vi "ImageAquisition.vi"() -> ()   [LabVIEW 2021]
uses:
  <vilib>/userdefined/High Color/IMAQdx.ctl
  <vilib>/vision/driver/IMAQdx.llb/IMAQdx Acquisition Mode.ctl
  <vilib>/vision/driver/IMAQdx.llb/IMAQdx Buffer Number Mode.ctl
  <vilib>/vision/driver/IMAQdx.llb/IMAQdx Camera Control Mode.ctl
  <vilib>/vision/driver/NI_Vision_Acquisition_Software.lvlib
panel:
  out "Image":T1(plugin-control)
  in  "Session In":T2="4kCam"
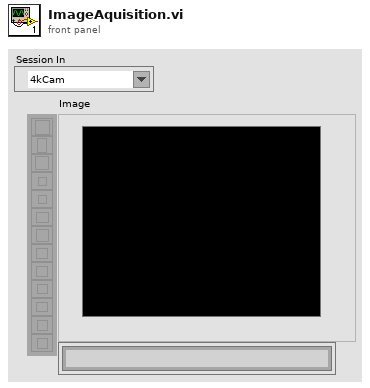
[diagram p1: front panel]
types:
  T1 = typedef "IMAQ Image.ctl" = refnum<image>
  T2 = typedef "IMAQdx.ctl" = refnum<k21>
  T3 = typedef "Image Type" = u32
  T4 = typedef "NI_Vision_Acquisition_Software.lvlib/IMAQdx Camera Control Mode.ctl" = enum32{"Controller", "Listener"}
  T5 = typedef "NI_Vision_Acquisition_Software.lvlib/IMAQdx Buffer Number Mode.ctl" = enum32{"Next", "Last", "Buffer Number", "Every", "Last New"}
  T6 = typedef "NI_Vision_Acquisition_Software.lvlib/IMAQdx Acquisition Mode.ctl" = enum32{"One Shot", "Continuous"}
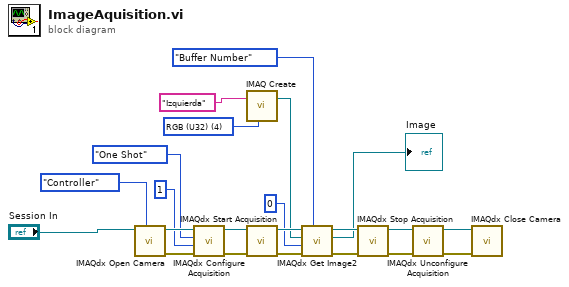
[diagram p0: block diagram]
diagram:
  w3 = T3 4 items=["Grayscale (U8)", "Grayscale (I16)", "Grayscale (SGL)", "Complex (CSG)", "RGB (U32)", "HSL (U32)", "RGB (U64)", "Grayscale (U16)"] ("Image Type")
  n1 = call <vilib>:"IMAQdx Open Camera.vi"("Camera Control Mode"=IMAQdx_Camera_Control_Mode."Controller", "Session In"="Session In") -> ("error out"=w20:errorcluster, "Session Out"=w22:T2)  [unwired: 8 in]
  n2 = call <vilib>:"IMAQdx Configure Acquisition.vi"("error in"=w20, "Number of Buffers"=u32 1, "Continuous?"=IMAQdx_Acquisition_Mode."One Shot", "Session In"=w22) -> ("error out"=w18:errorcluster, "Session Out"=w19:T2)  [unwired: 6 in]
  n3 = call "IMAQ Create"("Image Name"="Izquierda", "Image Type"=w3) -> ("New Image"=w2:T1)  [unwired: 3 in, 1 out]
  n4 = call <vilib>:"IMAQdx Start Acquisition.vi"("error in"=w18, "Session In"=w19) -> ("error out"=w16:errorcluster, "Session Out"=w17:T2)  [unwired: 8 in]
  n5 = call <vilib>:"IMAQdx Get Image2.vi"("Buffer Number Mode (Next)"=IMAQdx_Buffer_Number_Mode."Buffer Number", "error in"=w16, "Buffer Number In"=u32 0, "Image In"=w2, "Session In"=w17) -> ("error out"=w12:errorcluster, "Image Out"=→"Image":T1, "Session Out"=w13:T2)  [unwired: 3 in, 1 out]
  n6 = call <vilib>:"IMAQdx Stop Acquisition.vi"("error in"=w12, "Session In"=w13) -> ("error out"=w10:errorcluster, "Session Out"=w11:T2)  [unwired: 8 in]
  n7 = call <vilib>:"IMAQdx Unconfigure Acquisition.vi"("error in"=w10, "Session In"=w11) -> ("error out"=w8:errorcluster, "Session Out"=w9:T2)  [unwired: 8 in]
  n8 = call <vilib>:"IMAQdx Close Camera.vi"("error in"=w8, "Session In"=w9) -> ()  [unwired: 9 in, 1 out]
